vi "mult8x16.vi"(1 "y":i8, 2 "x":i16) -> (0 "x*y":i32)   [LabVIEW 2017]
doc: "Multiplies a 16-bit number by an 8-bit number to yield a 32-bit result."
uses:
  <vilib>/rvi/Arithmetic/AddSubMult/XNode/nirviSatArithmetic.xnode
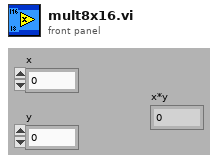
[diagram p1: front panel]
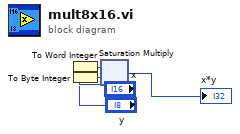
[diagram p0: block diagram]
diagram:
  n1 = To Word Integer(number="x") -> (16bit integer=w2:i16)
  n2 = To Byte Integer(number="y") -> (8bit integer=w1:i8)
  n3 = xnode "Saturation Multiply"("x"=w2, "y"=w1) -> ("x*y"=→"x*y":i32)
